vi "Write.vi"(8 "error in (no error)":errorcluster, 10 "write visa cmd buffer":string, 11 "PowerSupply_IT6333A in":refnum<class "PowerSupply_IT6333A.lvclass">) -> (0 "error out":errorcluster, 3 "PowerSupply_IT6333A out":refnum<class "PowerSupply_IT6333A.lvclass">)   [LabVIEW 2013, in "PowerSupply_IT6333A.lvclass"]
uses:
  PowerSupply_IT6333A.lvclass
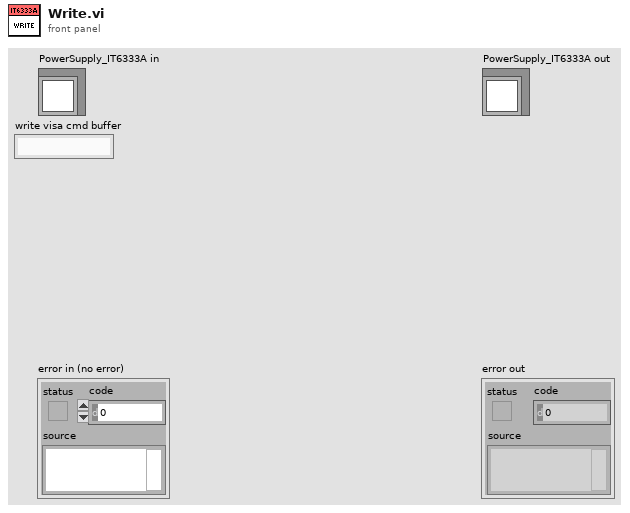
[diagram p1: front panel]
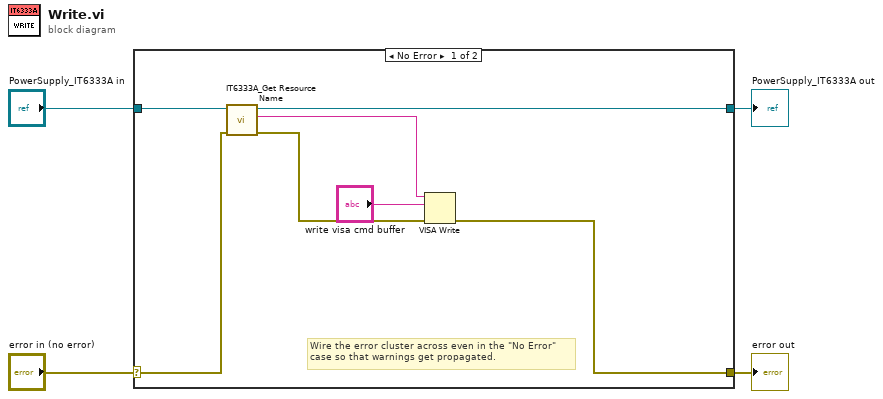
[diagram p0: block diagram]
diagram:
  n1 = case shown="No Error" "error in (no error)" {
    selector: "error in (no error)" -> [w8 w13]
    tunnel: [w7 w13] -> w3
    tunnel: [w10 w12] -> w1
    tunnel: "PowerSupply_IT6333A in" -> [w11 w12]
    frame No Error {
      # "Wire the error cluster across even in the \"No Error\"\ncase so that warnings get propagated."
      n2 = call-dynamic "IT6333A_Get Resource Name.vi"("error in (no error)"=w8, "PowerSupply_IT6333A in"=w11) -> ("error out"=w9:errorcluster, "Resource Name"=w6:string, "PowerSupply_IT6333A out"=w10:refnum<class "PowerSupply_IT6333A.lvclass">)  [unwired: 7 in]
      n3 = VISA Write(VISA resource name=w6, write buffer="write visa cmd buffer", error in (no error)=w9) -> (error out=w7:errorcluster)  [unwired: 2 out]
    }
    frame Error {
    }
  }
  "error out" <- w3
  "PowerSupply_IT6333A out" <- w1
